vi "Error Global.vi"(2 "Mode":enum16{"Read", "Write", "Clear Error"}(ring), 3 "Error In":errorcluster, 4 "Location In":string) -> (0 "Error Out":errorcluster, 1 "Location Out":string)   [LabVIEW 2019]
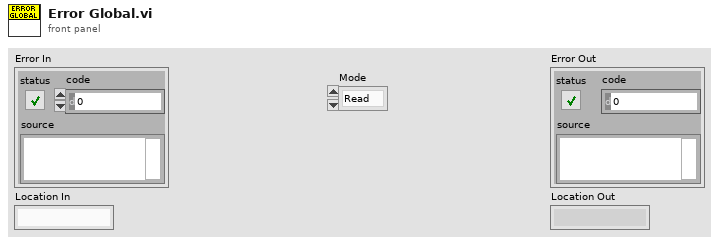
[diagram p1: front panel]
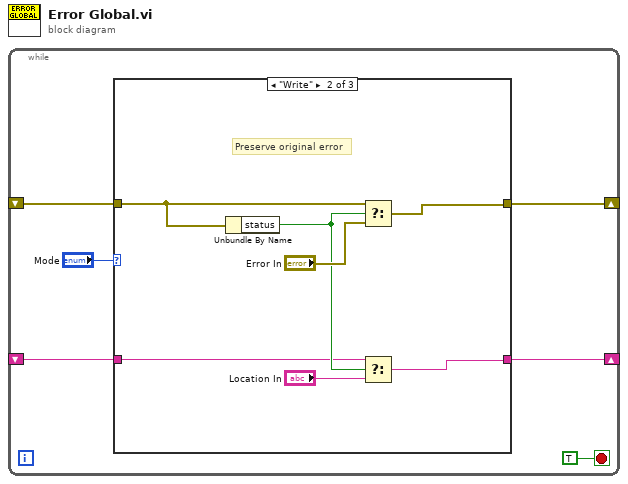
[diagram p0: block diagram]
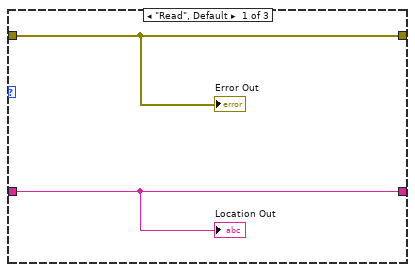
[diagram p2: hidden frame]
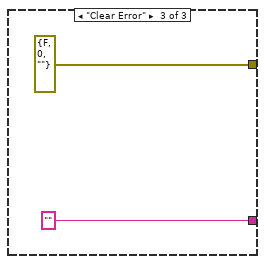
[diagram p3: hidden frame]
diagram:
  n1 = while {
    shift-right: [w4] -> _
    shift-left: _ -> [w3]
    shift-right: [w2] -> _
    shift-left: _ -> [w1]
    stop <- TRUE stop-if-true
    n2 = case shown="\"Write\"" "Mode" {
      tunnel: [w8 w13 errorcluster {"status"=FALSE, "code"=0, "source"=""} ("Error In")] -> w4
      tunnel: w3 -> [w8 w15 _]
      tunnel: [w7 w9 "" ("Location In")] -> w2
      tunnel: w1 -> [w7 w11 _]
      frame "Read", Default {
        "Error Out" <- w8
        "Location Out" <- w7
      }
      frame "Write" {
        # "Preserve original error"
        n3 = Unbundle By Name(w15) -> ("status"=w12:bool)
        n4 = Select(t=w15, s=w12, f="Error In") -> (s? t:f=w13:errorcluster)
        n5 = Select(t=w11, s=w12, f="Location In") -> (s? t:f=w9:string)
      }
      frame "Clear Error" {
      }
    }
  }
